vi "LSCI332ReadTemp.vi"(0 "VISA Rsrc":refnum<visa-resource-name>="GPIB0::12::INSTR", 5 "Activées":bool[](array[boolean]) caption="Entrés Activées", 11 "error in":errorcluster) -> (4 "Données":dbl[](array[numeric]), 15 "error out":errorcluster)   [LabVIEW 2019]
doc: "This VI querys the instrument for an inputs sensor reading in Celsius, Kelvin, and Sensor Units."
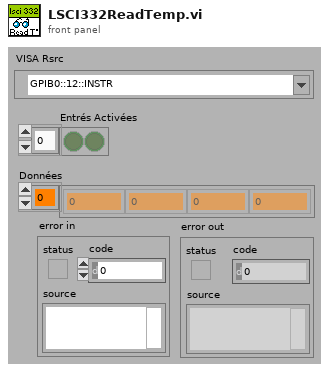
[diagram p1: front panel]
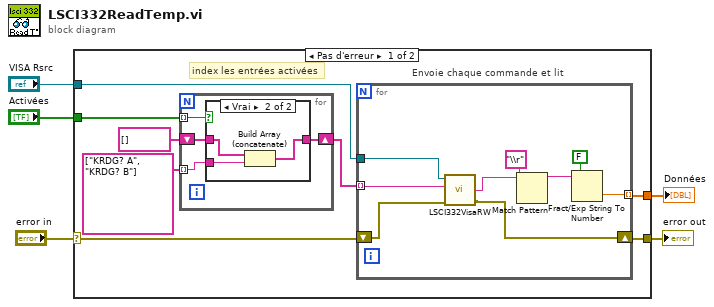
[diagram p0: block diagram]
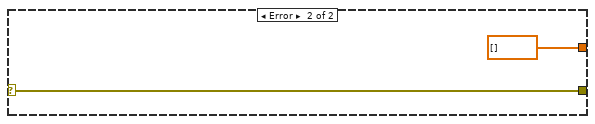
[diagram p3: hidden frame]
diagram:
  n1 = case shown="Pas d'erreur" "error in" {
    selector: "error in" -> [w10 w32]
    tunnel: [w13 w32] -> w5
    tunnel: "VISA Rsrc" -> [w12 _]
    tunnel: [w11 dbl[] []] -> w3
    tunnel: "Activées" -> [w8 _]
    frame No Error {
      # "index les entrées activées"
      # "Envoie chaque commande et lit"
      n2 = for {
        tunnel: string[] ["KRDG? A", "KRDG? B"] -> [w16] mode=indexing
        tunnel: w8 -> [w17] mode=indexing
        shift-right: [w15] -> w6
        shift-left: string[] [] -> [w14]
        n3 = case shown="Vrai" w17 {
          tunnel: w16 -> [_ w20]
          tunnel: [w18 w21] -> w15
          tunnel: w14 -> [w18 w19]
          frame False {
          }
          frame True {
            n4 = Build Array (concatenate)(w19, w20) -> (w21:string[])
          }
        }
      }
      n5 = for {
        tunnel: w6 -> [w25] mode=indexing
        shift-right: [w26] -> w13
        shift-left: w10 -> [w22]
        tunnel: w12 -> [w24]
        tunnel: [w30] -> w11 mode=indexing
        n6 = call <userlib>:"LSCI332VisaRW.vi"("error in (no error)"=w22, "ChaineCom"=w25, "VISA Rsrc"=w24) -> ("error out"=w26:errorcluster, "ChaineRep"=w23:string)  [unwired: 4 in, 2 out]
        n7 = Match Pattern(string=w23, regular expression="\\r") -> (before substring=w28:string)  [unwired: 1 in, 3 out]
        n8 = Fract/Exp String To Number(use system decimal point (T)=FALSE, string=w28) -> (number=w30:dbl)  [unwired: 2 in, 1 out]
      }
    }
    frame Error {
    }
  }
  "error out" <- w5
  "Données" <- w3
